vi "FPGA_PPG_application_example.vi"() -> ()   [LabVIEW 2014, in "NI-FPGA_PPG_Driver.lvlib"]
doc: "A simple application example for producing a few bit patterns with the FPGA.\n\nDietrich Beck, GSI Helmholtzzentrum fuer Schwerionenforschung, Germany"
uses:
  NI-FPGA_PPG_Driver.lvlib
  target/FPGA_target_state_type.ctl
panel:
  in  "mode":u8(ring) items=["once", "continous"]
  in  "stop":bool
  in  "command_lines 2":string[](array[string])=["$time::100000::1::0", "$time::100000::2::0", "$time::100000::4::0", "$time::100000::8::0", "$time::100000::16::0", "$time::100000::32::0", "$time::100000::64::0", "$time::100000::128::0", "$time::100000::256::0", "$time::100000::512::0", "$time::100000::1024::0", "$time::100000::2048::0", "$time::100000::4096::0", "$time::100000::8192::0", "$time::100000::16384::0", "$time::100000::32768::0", "$time::100000::65536::0", "$time::100000::131072::0", "$time::100000::262144::0", "$time::100000::524288::0", "$time::100000::1048576::0", "$time::100000::2097152::0", "$time::100000::4194304::0", "$time::100000::8388608::0", "$time::100000::16777216::0", "$time::100000::33554432::0", "$time::100000::67108864::0", "$time::100000::134217728::0", "$time::100000::268435456::0", "$time::100000::536870912::0", "$time::100000::1073741824::0", "$time::100000::2147483648::0", "$time::1000000::0::0", "$time::1000000::4294967295::0", "$time::1000000::0::4294967295", "$time::1000000::4294967295::0"]
  out "FPGA_state":T1
  in  "waitOnTrigger":bool
  out "Numeric":i32
  out "error out":errorcluster
  in  "command_lines":string[](array[string])=["$time::100000::1::0", "$time::100000::2::0", "$time::100000::4::0", "$time::100000::8::0", "$time::100000::16::0", "$time::100000::32::0", "$time::100000::64::0", "$time::100000::128::0", "$time::100000::256::0", "$time::100000::512::0", "$time::100000::1024::0", "$time::100000::2048::0", "$time::100000::4096::0", "$time::100000::8192::0", "$time::100000::16384::0", "$time::100000::32768::0", "$time::100000::65536::0", "$time::100000::131072::0", "$time::100000::262144::0", "$time::100000::524288::0", "$time::100000::1048576::0", "$time::100000::2097152::0", "$time::100000::4194304::0", "$time::100000::8388608::0", "$time::100000::16777216::0", "$time::100000::33554432::0", "$time::100000::67108864::0", "$time::100000::134217728::0", "$time::100000::268435456::0", "$time::100000::536870912::0", "$time::100000::1073741824::0", "$time::100000::2147483648::0", "$time::1000000::0::0", "$time::1000000::4294967295::0", "$time::1000000::0::4294967295", "$time::1000000::4294967295::0"]
  in  "resource_in":refnum<visa-resource-name>
  # "switch-on each channel on connector 0 for 100ms.\nThen, switch all channels on and off"
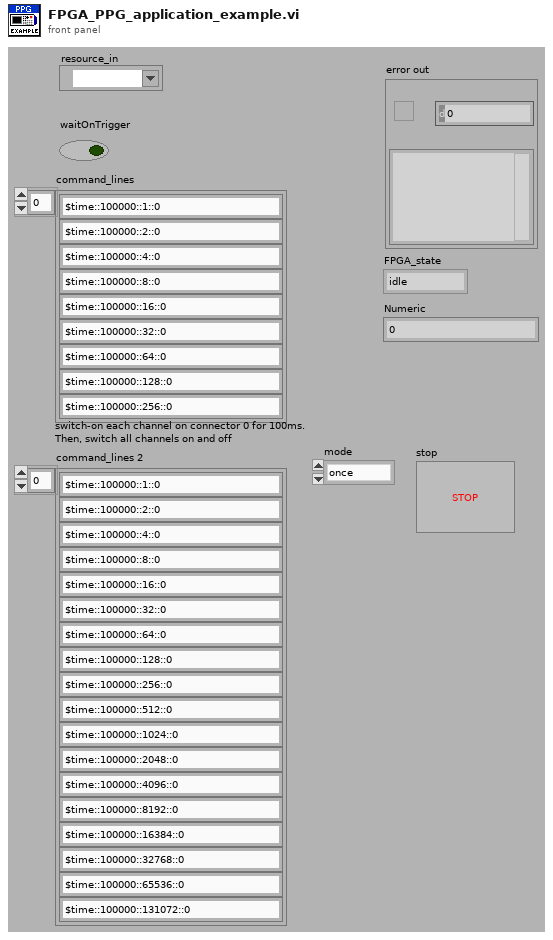
[diagram p1: front panel]
types:
  T1 = typedef "NI-FPGA_PPG_Driver.lvlib/FPGA_target_state_type.ctl" = enum16{"idle", "reset", "query", "load", "run", "stopped"}
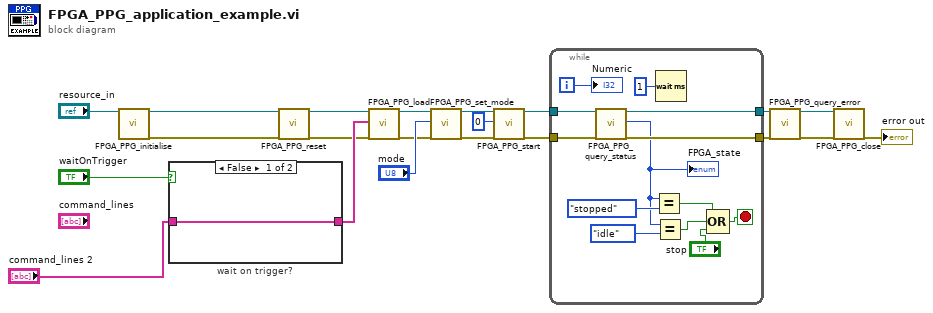
[diagram p0: block diagram]
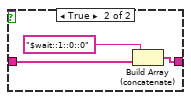
[diagram p2: hidden frame]
diagram:
  n1 = call "FPGA_PPG_initialise.vi"("resource_in"="resource_in") -> ("resource_out"=w5:refnum<visa-resource-name>, "error out"=w3:errorcluster)  [unwired: 16 in, 1 out]
  n2 = case "wait on trigger?" shown="False" "waitOnTrigger" {
    tunnel: "command_lines 2" -> [w22 w25]
    tunnel: [w22 w24] -> w8
    frame False {
    }
    frame True {
      n3 = Build Array (concatenate)("$wait::1::0::0", w25) -> (w24:string[])
    }
  }
  n4 = call "FPGA_PPG_reset.vi"("resource_in"=w5, "error in (no error)"=w3) -> ("resource_out"=w4:refnum<visa-resource-name>, "error out"=w2:errorcluster)  [unwired: 16 in]
  n5 = call "FPGA_PPG_load.vi"("resource_in"=w4, "command_lines"=w8, "error in (no error)"=w2) -> ("resource_out"=w6:refnum<visa-resource-name>, "error out"=w7:errorcluster)  [unwired: 15 in]
  n6 = call "FPGA_PPG_set_mode.vi"("resource_in"=w6, "mode"="mode", "error in (no error)"=w7) -> ("resource_out"=w12:refnum<visa-resource-name>, "error out"=w11:errorcluster)  [unwired: 15 in]
  n7 = call "FPGA_PPG_start.vi"("resource_in"=w12, "start_addr"=u32 0, "error in (no error)"=w11) -> ("resource_out"=w20:refnum<visa-resource-name>, "error out"=w19:errorcluster)  [unwired: 15 in]
  n8 = while {
    tunnel: w20 -> [w38]
    tunnel: w19 -> [w37]
    tunnel: [w36] -> w17
    tunnel: [w35] -> w16
    i -> [w34]
    stop <- w27 stop-if-true
    n9 = call "FPGA_PPG_query_status.vi"("resource_in"=w38, "error in (no error)"=w37) -> ("resource_out"=w35:refnum<visa-resource-name>, "FPGA_state"=w31:T1, "error out"=w36:errorcluster)  [unwired: 15 in]
    "FPGA_state" <- w31
    n10 = Equal?(x=w31, y=FPGA_target_state_type."stopped") -> (x = y?=w28:bool)
    n11 = Equal?(x=w31, y=FPGA_target_state_type."idle") -> (x = y?=w29:bool)
    n12 = Wait (ms)(milliseconds to wait=u32 1) -> ()  [unwired: 1 out]
    n13 = Compound Arithmetic op=OR(w28, w29, "stop") -> (w27:bool)
    "Numeric" <- w34
  }
  n14 = call "FPGA_PPG_query_error.vi"("resource_in"=w16, "error in (no error)"=w17) -> ("resource_out"=w14:refnum<visa-resource-name>, "error out"=w15:errorcluster)  [unwired: 16 in]
  n15 = call "FPGA_PPG_close.vi"("resource_in"=w14, "error in (no error)"=w15) -> ("error out"=→"error out":errorcluster)  [unwired: 17 in]
